vi "Teleop.vi"(10 "Match Info":T2={"Autonomous Elapsed Seconds"=0.0, "TeleOp Elapsed Seconds"=0.0, "Disabled Elapsed Seconds"=0.0, "Visited Autonomous"=FALSE, "Visited TeleOp"=FALSE, "Visited Disabled"=FALSE, "Autonomous Settings"={"Autonomous Style"=enum."Independent", "VI Refnum"=refnum}}, 11 "Call Context":T3) -> ()   [LabVIEW 2018]
doc: "This VI is called for each TeleOp packet received from the DS where the robot is not disabled. It is often used to read from the joysticks and update I/O or to update setpoints for timed control loops. It should complete and return within 20 milliseconds or it may miss DS packets."
uses:
  <vilib>/Rock Robotics/WPI/DriverStation/WPI_DriverStationDerivedRobotMode.ctl
  <vilib>/Rock Robotics/WPI/DriverStation/WPI_DriverStationMatch Info.ctl
  <vilib>/Rock Robotics/WPI/ThirdParty/Phoenix-LabVIEW/Motor Controller/Controls/CTRE_Phoenix_MotorControl_ControlMode.ctl
  <vilib>/Rock Robotics/Network Tables/NT Read Boolean.vi
  <vilib>/Rock Robotics/Network Tables/NT Read Number.vi
  <vilib>/Rock Robotics/WPI/Utilities/WPI_GetSetVariantRefNum.vi
  <vilib>/Rock Robotics/Network Tables/NT Write Boolean Array.vi
  <vilib>/Rock Robotics/Network Tables/NT Write Numeric Array.vi
  <vilib>/Rock Robotics/Network Tables/NT Write Boolean.vi
  <vilib>/Rock Robotics/Network Tables/NT Write Number.vi
  <vilib>/Rock Robotics/WPI/ThirdParty/Phoenix-LabVIEW/Motor Controller/Get/CTRE_Phoenix_MotorController_GetVoltage.vi
  <vilib>/Rock Robotics/WPI/ThirdParty/Phoenix-LabVIEW/Motor Controller/Get/CTRE_Phoenix_MotorController_GetSelectedSensorData.vi
  <vilib>/Rock Robotics/WPI/ThirdParty/Phoenix-LabVIEW/Motor Controller/Get/CTRE_Phoenix_MotorController_GetOutputCurrent_Enhanced.vi
  <vilib>/addons/control/pid/NI_PID_pid.lvlib
  Robot Global Data.vi
  <vilib>/addons/control/pid/pid.llb/PID (DBL).vi
panel:
  in  "Lift Position":i32=10000
  out "Button X 2":bool
  out "Button BACK 2":bool
  out "Button RT 2":bool
  out "Button LT 2":bool
  out "Button RB 2":bool
  out "Button LB 2":bool
  out "Button Y 2":bool
  out "Button B 2":bool
  out "Button A 2":bool
  in  "Right Max Acceleration (per 100ms)":i32=18000
  in  "Right Cruise Velocity (per 100 ms)":i32=20000
  out "Right Velocity per 100 ms":i32(graph)
  out "Right Position New 180":i32
  out "Right Position old":i32
  in  "Left Max Acceleration (per 100ms)":i32=18000
  in  "Left Cruise Velocity (per 100 ms)":i32=20000
  out "Left Velocity per 100 ms":i32(graph)
  out "Button Pressed?":bool
  out "Left Position New 180":i32
  out "Left Position old":i32
  out "Button X":bool
  out "Button BACK":bool
  out "Button RT":bool
  out "Button LT":bool
  out "Button RB":bool
  out "Button LB":bool
  out "Button Y":bool
  out "Button B":bool
  out "Button A":bool
  out "Wrist Position":i32=2000
  in  "Wrist Position":i32=10000 min=0 max=450000 step=50000
  out "Percent Output":dbl(graph)
  out "Position (Raw Sensor Units)":i32(graph)
  out "Velocity (Raw Sensor Units per 100 ms)":i32(graph)
  out "Elevator Position":i32=2000
  in  "Elevator Height":i32=10000 min=0 max=200000 step=10000
  out "Percent Output Elevator":dbl(graph)
  out "Position (Raw Sensor Units) 2":i32(graph)
  out "Velocity (Raw Sensor Units per 100 ms) 2":i32(graph)
  out "Output Current":dbl(graph)
  in  "Square Inputs":bool=TRUE
  in  "Gyro Rotation \nControl Enable?":bool
  in  "PID gains":T1={"proportional gain (Kc)"=0.02, "integral time (Ti, min)"=0.0, "derivative time (Td, min)"=0.0}
  in  "output range":cluster{"output high":dbl, "output low":dbl}={"output high"=0.6, "output low"=-0.6}
  out "Sample Slider 0":dbl(slide) scale=0.0..5.0
  out "Sample Boolean 1":bool
  out "Sample Boolean 0":bool
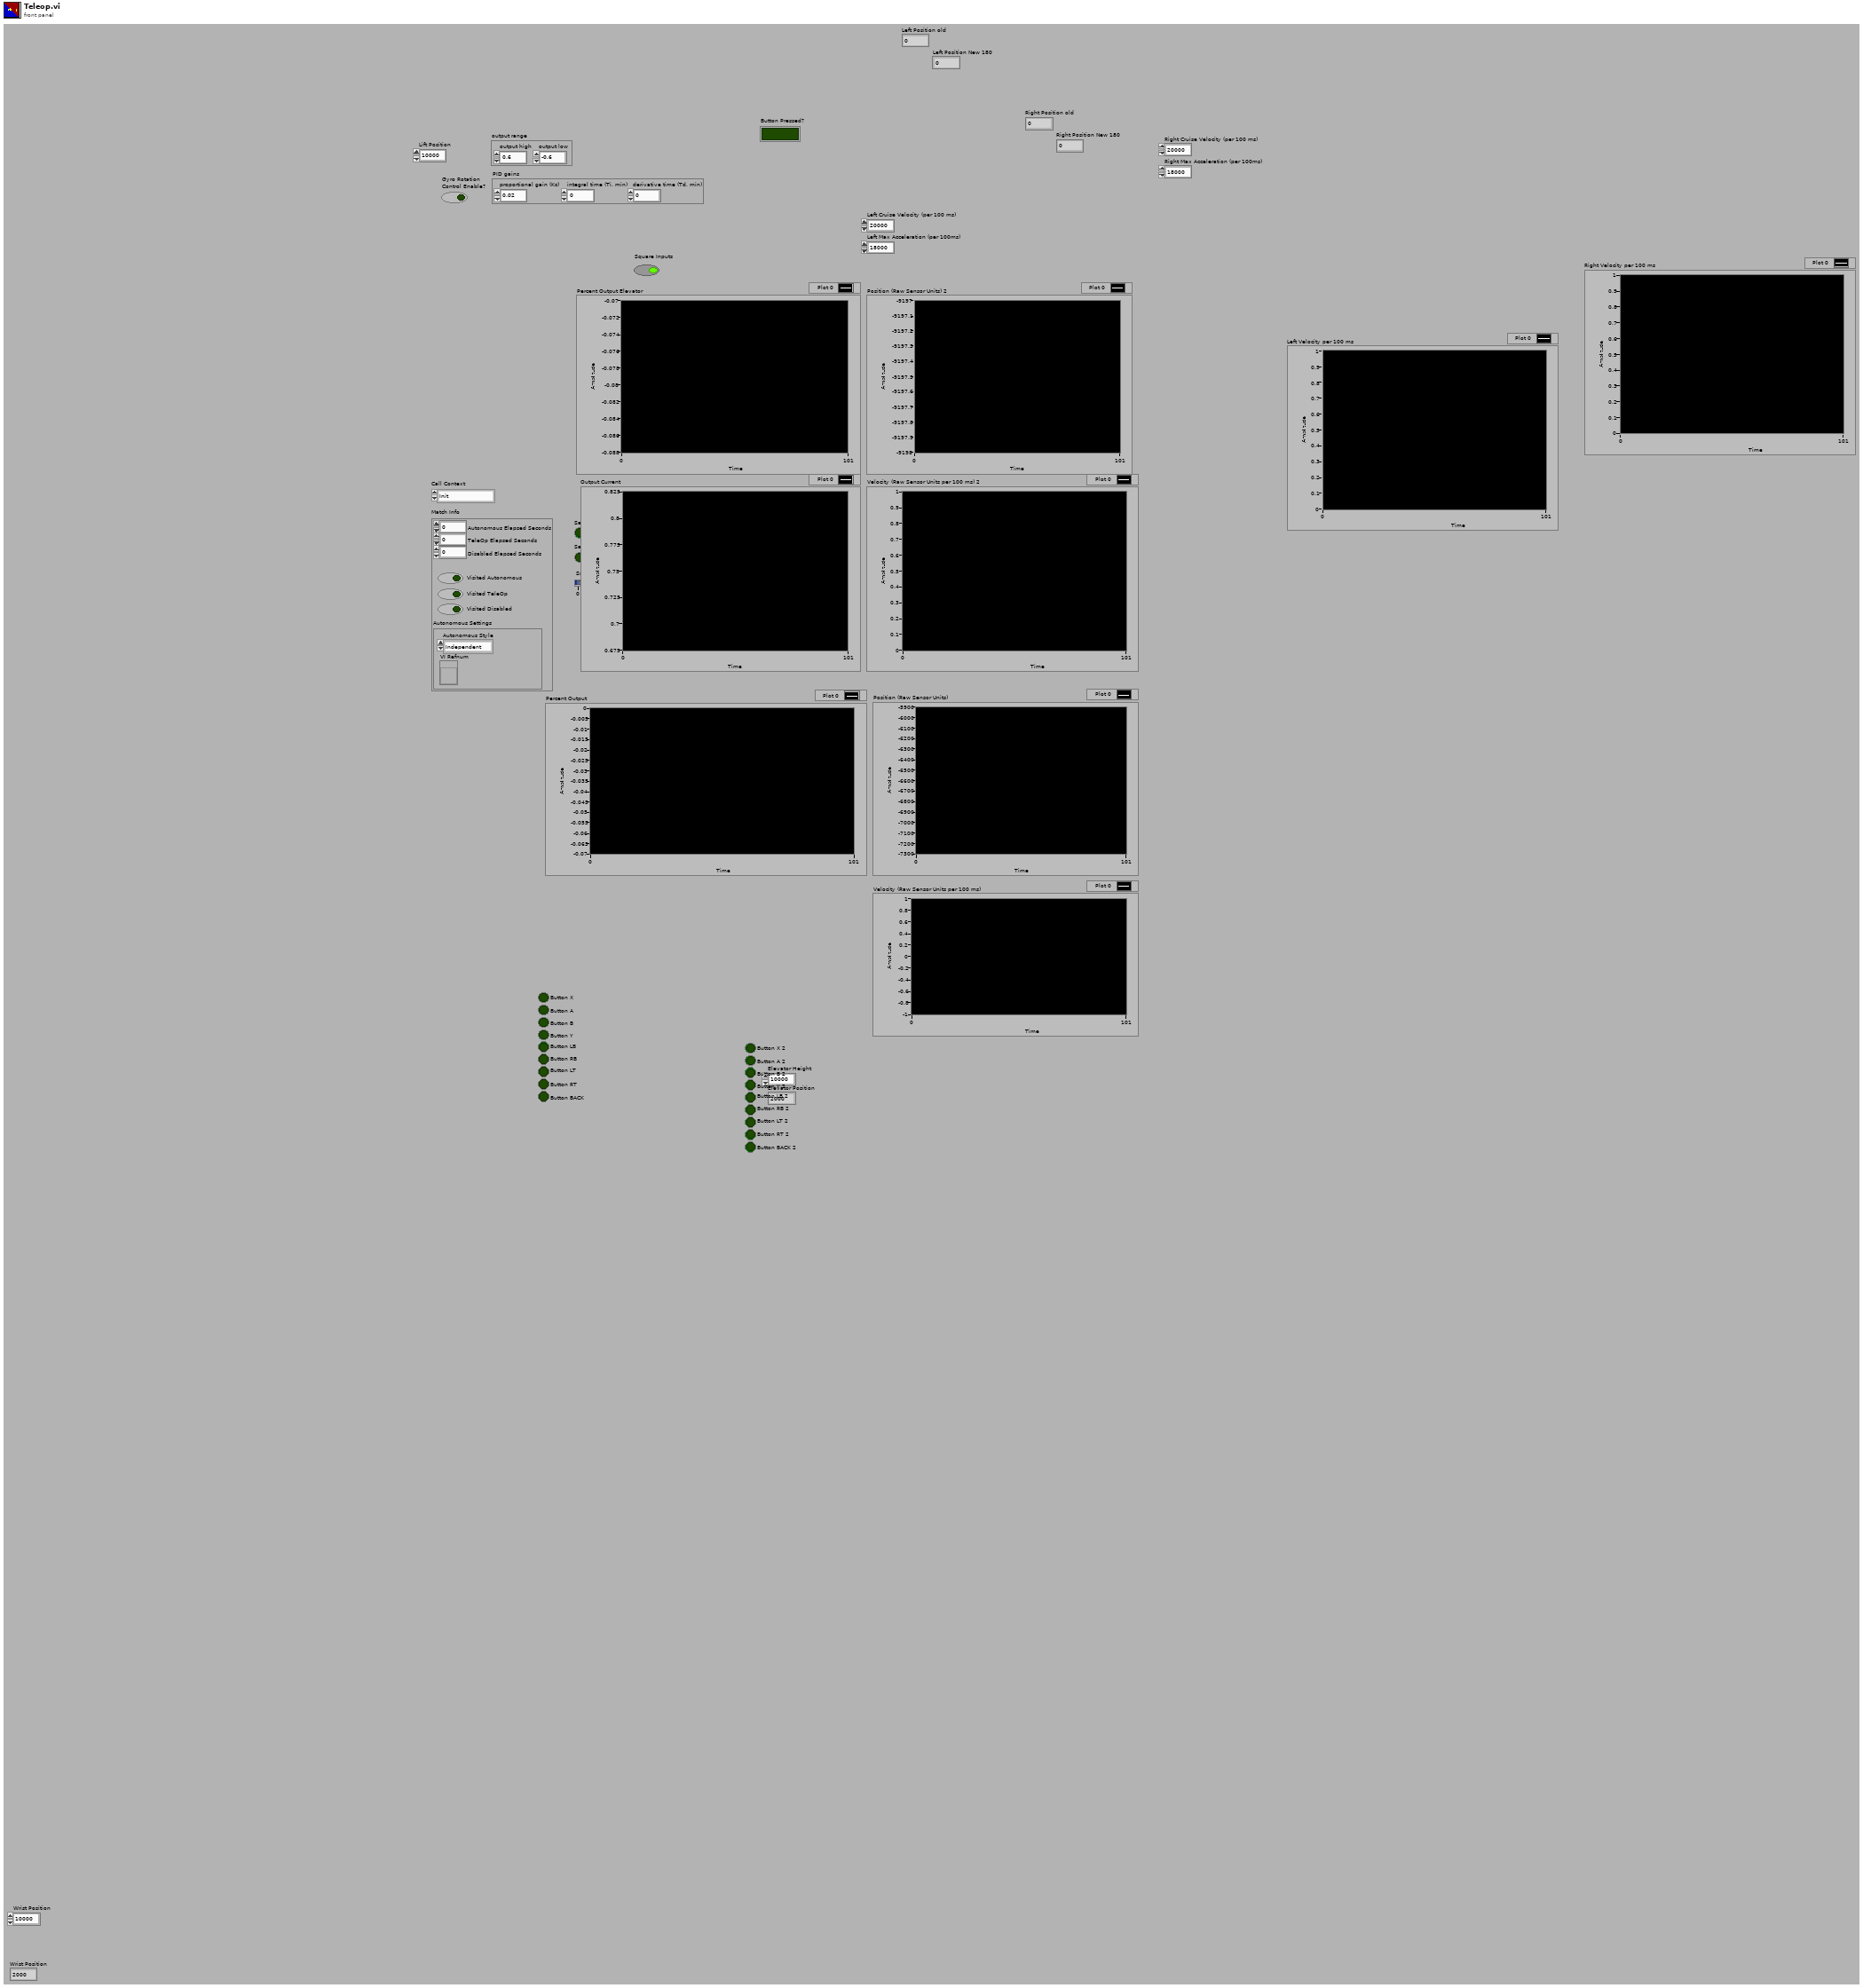
[diagram p1: front panel]
types:
  T1 = cluster{"proportional gain (Kc)":dbl, "integral time (Ti, min)":dbl, "derivative time (Td, min)":dbl}
  T2 = typedef "WPI_DriverStationMatch Info.ctl" = cluster{"Autonomous Elapsed Seconds":dbl, "TeleOp Elapsed Seconds":dbl, "Disabled Elapsed Seconds":dbl, "Visited Autonomous":bool, "Visited TeleOp":bool, "Visited Disabled":bool, "Autonomous Settings":cluster{"Autonomous Style":enum16{"Iterative", "Independent"}, "VI Refnum":refnum<vi>}}
  T3 = typedef "WPI_DriverStationDerivedRobotMode.ctl" = enum16{"Init", "Execute", "Stop"}
  T4 = typedef "CTRE_Phoenix_MotorControl_ControlMode.ctl" = u16
  T5 = typedef "WPI_JoystickDevRef.ctl" = cluster{"Device":T6}
  T6 = typedef "WPI_JoystickDeviceEnum.ctl" = enum16{"USB 0", "USB 1", "USB 2", "USB 3", "USB 4", "USB 5"}
  T7 = cluster{"Buttons[0]":bool, "Buttons[1]":bool, "Buttons[2]":bool, "Buttons[3]":bool, "Buttons[4]":bool, "Buttons[5]":bool, "Buttons[6]":bool, "Buttons[7]":bool, "Buttons[8]":bool}
  T8 = typedef "WPI_GyroDevRef.ctl" = cluster{"DevStatus":errorcluster, "Analog Channel":T9, "Gain (VoltsPerDegree/Second)":dbl, "Gyro Type":enum16{"Analog", "XRS450"}, "Handle":i32, "SPI Bus":T10, "Device Found":bool, "Sample Rate":dbl, "Calibrate On Open":bool, "Offset":dbl}
  T9 = typedef "FPGA_AIChannel.ctl" = enum8{"AI 0", "AI 1", "AI 2", "AI 3", "AI MXP 0", "AI MXP 1", "AI MXP 2", "AI MXP 3", "Invalid"}
  T10 = typedef "spi_bus.ctl" = enum16{"SPI On-Board, CS0", "SPI On-Board, CS1", "SPI On-Board, CS2", "SPI On-Board, CS3", "SPI MXP", "Invalid"}
  T11 = typedef "WPI_MotorControlDeviceRef.ctl" = cluster{"DeviceStatus":errorcluster, "Type":T12, "PWM":cluster{"PWM Channel":T13, "DeadBand":T14}, "CAN":cluster{"Device Number":u8, "SetOutput VI Ref":variant, "GetOutput VI Ref":variant, "Enable VI Ref":variant, "Disable VI Ref":variant, "Data":variant}, "Invert":bool, "DIO PWM":cluster{"PWM \"Enable\" Channel":T13, "DIOChannel":T15, "PWM Rate":dbl}}
  T12 = typedef "WPI_MotorControlType.ctl" = enum16{"PWM", "CAN", "DIO PWM"}
  T13 = typedef "FPGA_DIOPWMChannel.ctl" = enum8{"PWM 0", "PWM 1", "PWM 2", "PWM 3", "PWM 4", "PWM 5", "PWM 6", "PWM 7", "PWM 8", "PWM 9", "PWM MXP 0", "PWM MXP 1", "PWM MXP 2", "PWM MXP 3", "PWM MXP 4", "PWM MXP 5", "PWM MXP 6", "PWM MXP 7", "PWM MXP 8", "PWM MXP 9", "Invalid"}
  T14 = typedef "WPI_PWMDeadband.ctl" = cluster{"Name":string, "maxPositivePwm":i32, "minPositivePwm":i32, "centerPwm":i32, "maxNegativePwm":i32, "minNegativePwm":i32, "angularRange":u16}
  T15 = typedef "FPGA_DIOChannel.ctl" = enum8{"DIO 0", "DIO 1", "DIO 2", "DIO 3", "DIO 4", "DIO 5", "DIO 6", "DIO 7", "DIO 8", "DIO 9", "DIO MXP 0", "DIO MXP 1", "DIO MXP 2", "DIO MXP 3", "DIO MXP 4", "DIO MXP 5", "DIO MXP 6", "DIO MXP 7", "DIO MXP 8", "DIO MXP 9", "DIO MXP 10", "DIO MXP 11", "DIO MXP 12", "DIO MXP 13", "DIO MXP 14", "DIO MXP 15", "SPI Port CS1", "SPI Port CS2", "SPI Port CS3", "SPI Port MISO", "SPI Port MOSI", "Invalid"}
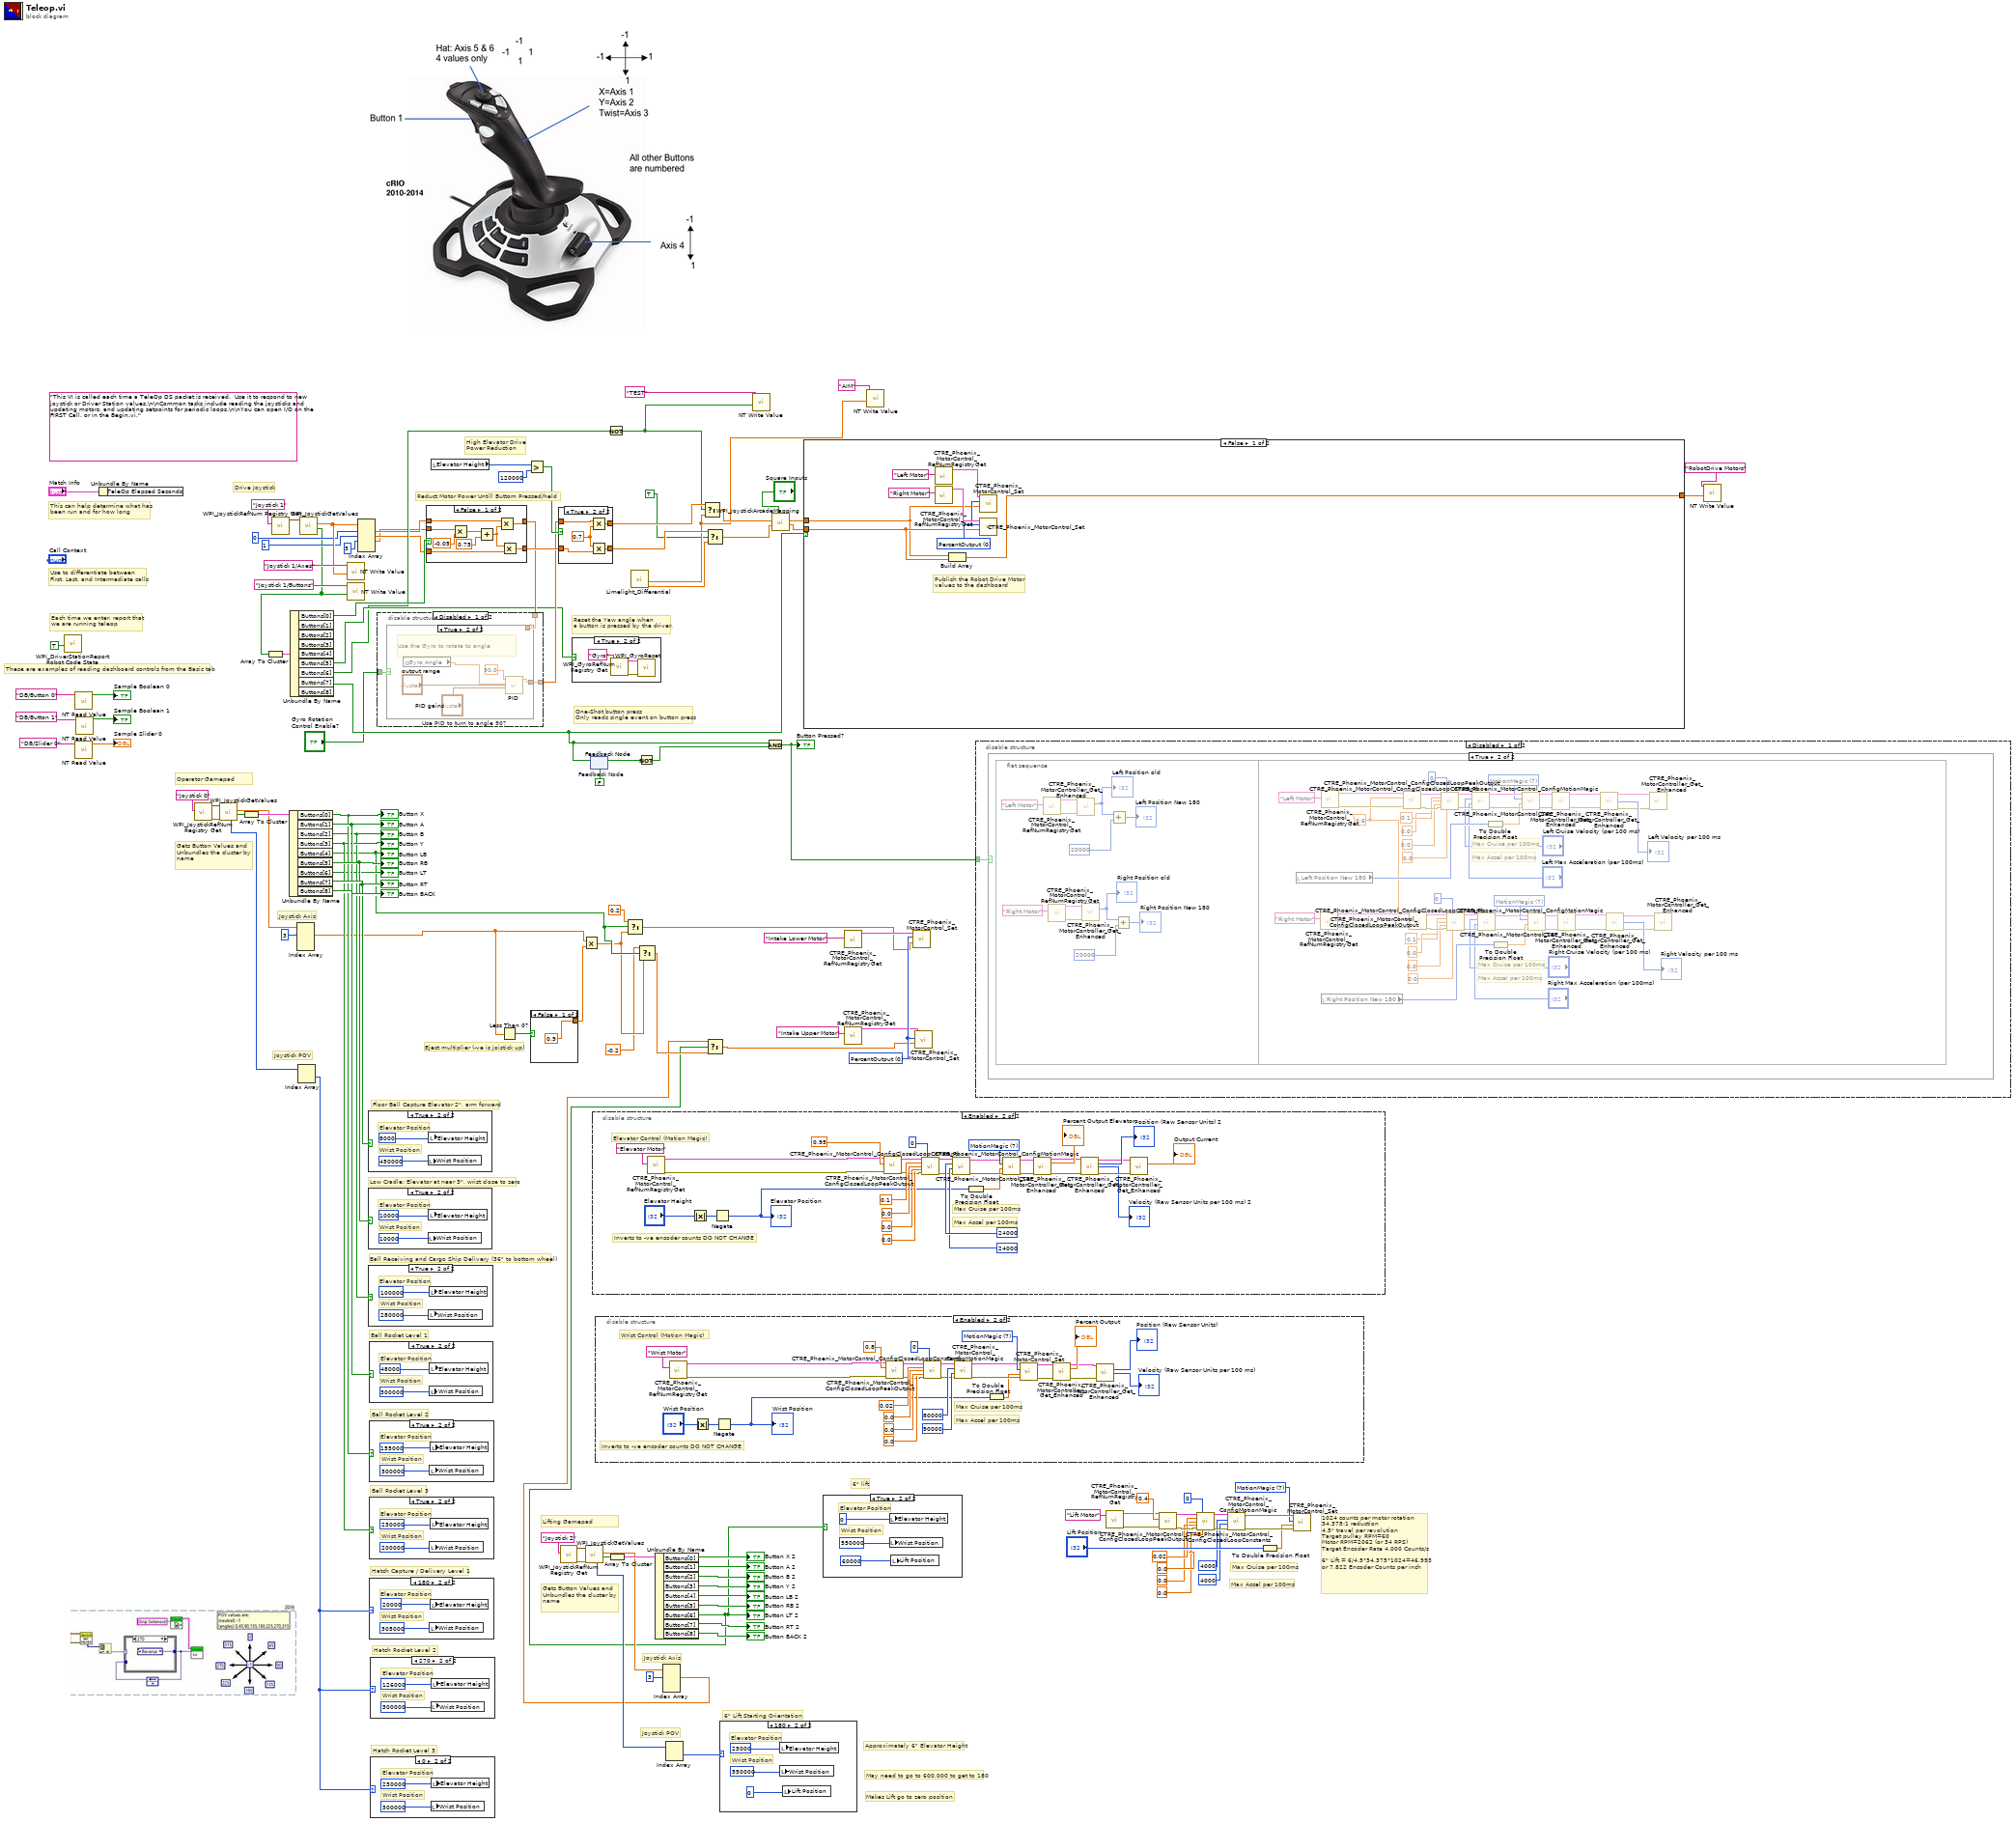
[diagram p0: block diagram]
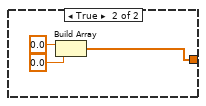
[diagram p8: hidden frame]
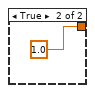
[diagram p9: hidden frame]
diagram:
  w4 = T4 7 items=["PercentOutput"=0, "Position"=1, "Velocity"=2, "Current"=3, "Follower"=5, "MotionProfile"=6, "MotionMagic"=7, "MotionProfileArc"=10, "Disabled"=15] ("Wrist Control Mode")
  w74 = T4 0 items=["PercentOutput"=0, "Position"=1, "Velocity"=2, "Current"=3, "Follower"=5, "MotionProfile"=6, "MotionMagic"=7, "MotionProfileArc"=10, "Disabled"=15] ("Control Mode")
  (unwired) "This VI is called each time a TeleOp DS packet is received.  Use it to respond to new joystick or Driver Station values.\n\nCommon tasks include reading the joysticks and updating motors, and updating setpoints for periodic loops.\n\nYou can open I/O on the FIRST Call, or in the Begin.vi."
  # "6\" lift"
  # "1024 counts per motor rotation\n34.375:1 reduction\n4.5\" travel per revolution\nTarget pulley RPM=60\nMotor RPM=2062 (or 34 RPS)\nTarget Encoder Rate 4,000 Counts/s\n\n6\" Lift = 6/4.5*34.375*1024=46,993\nor 7,822 Encoder Counts per inch"
  # "Max Accel per 100ms"
  # "Max Cruise per 100ms"
  # "Makes Lift go to zero position"
  # "Approximately 6\" Elevator Height"
  # "May need to go to 600,000 to get to 180"
  # "6\" Lift Starting Orientation"
  # "Joystick POV"
  # "Joystick Axis"
  # "Lifting Gamepad"
  # "Gets Button Values and Unbundles the cluster by name"
  # "One-Shot button press \nOnly reads single event on button press"
  # "Eject multiplier (-ve is joistick up)"
  # "Ball Rocket Level 3"
  # "Hatch Rocket Level 2"
  # "Joystick POV"
  # "Hatch Rocket Level 3"
  # "Hatch Capture / Delivery Level 1"
  # "Ball Rocket Level 2"
  # "Ball Rocket Level 1"
  # "Ball Receiving and Cargo Ship Delivery (36\" to bottom wheel)"
  # "Low Cradle: Elevator at near 3\", wrist close to zero"
  # "Floor Ball Capture Elevator 2\", arm forward"
  # "Joystick Axis"
  # "Operator Gamepad"
  # "Gets Button Values and Unbundles the cluster by name"
  # "Reset the Yaw angle when \na button is pressed by the driver."
  # "High Elevator Drive \nPower Reduction"
  # "Reduct Motor Power Untill Buttom Pressed/held"
  # "Drive Joystick"
  # "These are examples of reading dashboard controls from the Basic tab"
  # "Each time we enter, report that\nwe are running teleop"
  # "Use to differentiate between\nFirst, Last, and Intermediate calls"
  # "This can help determine what has\nbeen run and for how long"
  n1 = call <vilib>:"WPI_DriverStationReport Robot Code State.vi"("TeleOp"=TRUE ("Autonomous")) -> ()  [unwired: 10 in, 1 out]
  n2 = call-poly <vilib>:"NT Read Value.vi"("Name"="DB/Button 0" ("refnum name")) -> ("Boolean"=→"Sample Boolean 0":bool)  [unwired: 9 in, 1 out]
  n3 = call-poly <vilib>:"NT Read Value.vi"("Name"="DB/Slider 0" ("refnum name")) -> ("Numeric"=→"Sample Slider 0":dbl)  [unwired: 9 in, 1 out]
  n4 = call-poly <vilib>:"NT Read Value.vi"("Name"="DB/Button 1" ("refnum name")) -> ("Boolean"=→"Sample Boolean 1":bool)  [unwired: 9 in, 1 out]
  n5 = Unbundle By Name("Match Info") -> ()  [unwired: 1 out]
  n6 = call <vilib>:"WPI_JoystickRefNum Registry Get.vi"("refnum name"="Joystick 0") -> ("error out"=w87:errorcluster, "JoystickDevRef"=w88:T5)  [unwired: 1 in, 8 out]
  n7 = call <vilib>:"WPI_JoystickGetValues.vi"("error in (no error)"=w87, "JoystickDevRef"=w88) -> ("Buttons"=w84:bool[], "Axes"=w86:dbl[], "POVs"=w85:i16[])  [unwired: 5 in, 2 out]
  n8 = Array To Cluster(array=w84) -> (cluster=w94:T7)
  n9 = call <vilib>:"WPI_JoystickRefNum Registry Get.vi"("refnum name"="Joystick 1") -> ("JoystickDevRef"=w113:T5)  [unwired: 1 in, 9 out]
  n10 = Unbundle By Name(w94) -> ("Buttons[0]"=w82:bool, "Buttons[1]"=w83:bool, "Buttons[2]"=w80:bool, "Buttons[3]"=w81:bool, "Buttons[4]"=w77:bool, "Buttons[5]"=w90:bool, "Buttons[6]"=→"Button LT":bool, "Buttons[7]"=w91:bool, "Buttons[8]"=→"Button BACK":bool)
  "Button A" <- w83
  "Button B" <- w80
  "Button Y" <- w81
  "Button LB" <- w77
  "Button RB" <- w90
  "Button RT" <- w91
  "Button X" <- w82
  n11 = Index Array(array=w86, index #1=3 ("index")) -> (element #1=w78:dbl)  [unwired: 3 in, 3 out]
  n12 = Index Array(array=w85) -> (element #1=w89:i16)  [unwired: 2 in, 1 out]
  n13 = call <vilib>:"WPI_JoystickGetValues.vi"("JoystickDevRef"=w113) -> ("Buttons"=w102:bool[], "Axes"=w110:dbl[])  [unwired: 6 in, 3 out]
  n14 = Array To Cluster(array=w102) -> (cluster=w104:T7)
  n15 = Unbundle By Name(w104) -> ("Buttons[0]"=w103:bool, "Buttons[5]"=w99:bool, "Buttons[6]"=w54:bool, "Buttons[7]"=w61:bool)  [unwired: 5 out]
  n16 = call-poly <vilib>:"NT Write Value.vi"("Numeric Array"=w110, "Name"="Joystick 1/Axes") -> ()  [unwired: 9 in, 1 out]
  n17 = call-poly <vilib>:"NT Write Value.vi"("Boolean Array"=w102, "Name"="Joystick 1/Buttons") -> ()  [unwired: 9 in, 1 out]
  n18 = Index Array(array=w110, index #1=0 ("index"), index #2=1 ("index"), index #3=3 ("index")) -> (element #1=w53:dbl, element #2=w52:dbl, element #3=w42:dbl)  [unwired: 2 in, 2 out]
  n19 = case shown="True" w91 {
    frame False {
    }
    frame True {
      # "Wrist Position"
      # "Elevator Position"
      n20 = local write "Wrist Position"(450000) -> ()
      n21 = local write "Elevator Height"(8000) -> ()
    }
  }
  n22 = case shown="True" w90 {
    frame False {
    }
    frame True {
      # "Wrist Position"
      # "Elevator Position"
      n23 = local write "Wrist Position"(10000) -> ()
      n24 = local write "Elevator Height"(10000) -> ()
    }
  }
  n25 = case shown="True" w80 {
    frame False {
    }
    frame True {
      # "Wrist Position"
      # "Elevator Position"
      n26 = local write "Wrist Position"(280000) -> ()
      n27 = local write "Elevator Height"(100000) -> ()
    }
  }
  n28 = case shown="True" w83 {
    frame False {
    }
    frame True {
      # "Wrist Position"
      # "Elevator Position"
      n29 = local write "Wrist Position"(300000) -> ()
      n30 = local write "Elevator Height"(48000) -> ()
    }
  }
  n31 = case shown="True" w82 {
    frame False {
    }
    frame True {
      # "Wrist Position"
      # "Elevator Position"
      n32 = local write "Wrist Position"(300000) -> ()
      n33 = local write "Elevator Height"(155000) -> ()
    }
  }
  n34 = case shown="True" w81 {
    frame False {
    }
    frame True {
      # "Wrist Position"
      # "Elevator Position"
      n35 = local write "Wrist Position"(200000) -> ()
      n36 = local write "Elevator Height"(230000) -> ()
    }
  }
  n37 = case shown="180" w89 {
    frame -1, Default {
    }
    frame 180 {
      # "Wrist Position"
      # "Elevator Position"
      n38 = local write "Wrist Position"(305000) -> ()
      n39 = local write "Elevator Height"(20000) -> ()
    }
  }
  n40 = case shown="270" w89 {
    frame -1, Default {
    }
    frame 270 {
      # "Wrist Position"
      # "Elevator Position"
      n41 = local write "Wrist Position"(300000) -> ()
      n42 = local write "Elevator Height"(126000) -> ()
    }
  }
  n43 = case shown="0" w89 {
    frame -1, Default {
    }
    frame 0 {
      # "Wrist Position"
      # "Elevator Position"
      n44 = local write "Wrist Position"(300000) -> ()
      n45 = local write "Elevator Height"(230000) -> ()
    }
  }
  n46 = case shown="False" w103 {
    tunnel: [w148 w154] -> w101
    tunnel: [w149 w152] -> w105
    tunnel: w53 -> [w147 w151]
    tunnel: w52 -> [w146 w150]
    tunnel: w42 -> [w145 _]
    frame False {
      n47 = Multiply(x=w145, y=-0.05 ("drive multiplyer")) -> (x*y=w143:dbl)
      n48 = Add(x=w143, y=0.75 ("drive multiplyer")) -> (x+y=w141:dbl)
      n49 = Multiply(x=w147, y=w141) -> (x*y=w148:dbl)
      n50 = Multiply(x=w141, y=w146) -> (x*y=w149:dbl)
    }
    frame True {
      w153 = 1.0
      n51 = Multiply(x=w151, y=w153) -> (x*y=w154:dbl)
      n52 = Multiply(x=w153, y=w150) -> (x*y=w152:dbl)
    }
  }
  n53 = disable-structure shown="Disabled" {
    disable-tunnel: w101 -> [w157 _]
    disable-tunnel: [w156 _] -> w100
    disable-tunnel: "Gyro Rotation \nControl Enable?" -> [w155 _]
    frame Disabled {
      n54 = case "Use PID to turn to angle 90?" shown="True" w155 {
        tunnel: [w158 w160] -> w156
        tunnel: w157 -> [w158 _]
        frame False {
        }
        frame True {
          # "Use the Gyro to rotate to angle"
          n55 = global read "Robot Global Data.vi" "Gyro Angle"() -> (w159:dbl)
          n56 = call-poly <vilib>:"PID.vi"("output range"="output range", "PID gains"="PID gains", "process variable"=w159, "setpoint"=90.0) -> ("output"=w160:dbl)  [unwired: 6 in, 1 out]
        }
      }
    }
    frame Enabled {
    }
  }
  n57 = local read "Elevator Height"() -> (w65:i32)
  n58 = Less Than 0?(x=w78) -> (x < 0?=w66:bool)
  n59 = Greater?(x=w65, y=120000) -> (0:w106:bool)
  n60 = case shown="False" w66 {
    tunnel: [0.9 1.0] -> w70
    frame False {
    }
    frame True {
    }
  }
  n61 = case shown="True" w106 {
    tunnel: w100 -> [w167 w171]
    tunnel: w105 -> [w166 w170]
    tunnel: [w167 w169] -> w47
    tunnel: [w166 w168] -> w48
    frame False {
    }
    frame True {
      w172 = 0.7
      n62 = Multiply(x=w171, y=w172) -> (x*y=w169:dbl)
      n63 = Multiply(x=w172, y=w170) -> (x*y=w168:dbl)
    }
  }
  n64 = call <vilib>:"WPI_JoystickRefNum Registry Get.vi"("refnum name"="Joystick 2") -> ("error out"=w35:errorcluster, "JoystickDevRef"=w36:T5)  [unwired: 1 in, 8 out]
  n65 = case shown="True" w99 {
    frame False {
    }
    frame True {
      n66 = call <vilib>:"WPI_GyroRefNum Registry Get.vi"("refnum name"="Gyro") -> ("error out"=w173:errorcluster, "GyroDevRef"=w174:T8)  [unwired: 9 in]
      n67 = call <vilib>:"WPI_GyroReset.vi"("error in"=w173, "GyroDevRef"=w174) -> ()  [unwired: 8 in, 2 out]
    }
  }
  n68 = Multiply(x=w78, y=w70) -> (x*y=w71:dbl)
  n69 = call <vilib>:"WPI_JoystickGetValues.vi"("error in (no error)"=w35, "JoystickDevRef"=w36) -> ("Buttons"=w33:bool[], "Axes"=w34:dbl[], "POVs"=w27:i16[])  [unwired: 5 in, 2 out]
  n70 = feedback #1 "Feedback Node"(FALSE ("Button In")) -> (w64:bool)
  n71 = feedback-in #1(w61) -> ()
  n72 = disable-structure shown="Enabled" {
    frame Disabled {
    }
    frame Enabled {
      w196 = T4 7 items=["PercentOutput"=0, "Position"=1, "Velocity"=2, "Current"=3, "Follower"=5, "MotionProfile"=6, "MotionMagic"=7, "MotionProfileArc"=10, "Disabled"=15] ("Elevator Control Mode")
      # "Max Accel per 100ms"
      # "Max Cruise per 100ms"
      # "Inverts to -ve encoder counts DO NOT CHANGE"
      # "Elevator Control (Motion Magic)"
      n73 = call <vilib>:"CTRE_Phoenix_MotorControl_RefNumRegistryGet.vi"("refnum name"="Elevator Motor") -> ("error out"=w186:errorcluster, "PhoenixMotorControlDevRef"=w187:T11)  [unwired: 9 in]
      n74 = Absolute Value(x="Elevator Height") -> (abs(x)=w195:i32)
      n75 = Negate(x=w195) -> (-x=w188:i32)
      "Elevator Position" <- w188
      n76 = call <vilib>:"CTRE_Phoenix_MotorControl_ConfigClosedLoopPeakOutput.vi"("error in (no error)"=w186, "peakOutput"=0.95 ("Peak Elevator Power"), "PhoenixMotorControlDevRef"=w187) -> ("error out"=w192:errorcluster, "PhoenixMotorControlDevRef"=w205:T11)  [unwired: 7 in]
      n77 = call <vilib>:"CTRE_Phoenix_MotorControl_ConfigClosedLoopConstants.vi"("PhoenixMotorControlDevRef"=w205, "slotIdx"=0, "P"=0.1 ("P 2"), "I"=0.0 ("I 2"), "D"=0.0 ("D 2"), "error in (no error)"=w192, "F"=0.0 ("F 2")) -> ("PhoenixMotorControlDevRef"=w200:T11, "error out"=w191:errorcluster)  [unwired: 7 in]
      n78 = call <vilib>:"CTRE_Phoenix_MotorControl_ConfigMotionMagic.vi"("error in (no error)"=w191, "Acceleration"=24000 ("Elevator Max Acceleration (per 100ms)"), "Cruise Velocity"=24000 ("Elevator Cruise Velocity (per 100 ms)"), "PhoenixMotorControlDevRef"=w200) -> ("error out"=w190:errorcluster, "PhoenixMotorControlDevRef"=w193:T11)  [unwired: 6 in]
      n79 = To Double Precision Float(number=w188) -> (double precision float=w189:dbl)
      n80 = call <vilib>:"CTRE_Phoenix_MotorControl_Set.vi"("error in (no error)"=w190, "Output"=w189, "Control Mode"=w196, "PhoenixMotorControlDevRef"=w193) -> ("error out"=w184:errorcluster, "PhoenixMotorControlDevRef"=w185:T11)  [unwired: 6 in]
      n81 = call-poly <vilib>:"CTRE_Phoenix_MotorController_Get_Enhanced.vi"("PhoenixMotorControlDevRef"=w185, "error in"=w184) -> ("PhoenixMotorControlDevRef"=w182:T11, "Percent Output"=→"Percent Output Elevator":dbl, "error out"=w181:errorcluster)  [unwired: 9 in, 2 out]
      n82 = call-poly <vilib>:"CTRE_Phoenix_MotorController_Get_Enhanced.vi"("PhoenixMotorControlDevRef"=w182, "error in"=w181) -> ("PhoenixMotorControlDevRef"=w179:T11, "Position (Raw Sensor Units)"=→"Position (Raw Sensor Units) 2":i32, "Velocity (Raw Sensor Units per 100 ms)"=→"Velocity (Raw Sensor Units per 100 ms) 2":i32, "error out"=w178:errorcluster)  [unwired: 10 in]
      n83 = call-poly <vilib>:"CTRE_Phoenix_MotorController_Get_Enhanced.vi"("PhoenixMotorControlDevRef"=w179, "error in"=w178) -> ("Output Current"=→"Output Current":dbl)  [unwired: 11 in, 2 out]
    }
  }
  n84 = disable-structure shown="Enabled" {
    frame Disabled {
    }
    frame Enabled {
      w225 = T4 7 items=["PercentOutput"=0, "Position"=1, "Velocity"=2, "Current"=3, "Follower"=5, "MotionProfile"=6, "MotionMagic"=7, "MotionProfileArc"=10, "Disabled"=15] ("Wrist Control Mode")
      # "Max Accel per 100ms"
      # "Max Cruise per 100ms"
      # "Inverts to -ve encoder counts DO NOT CHANGE"
      # "Wrist Control (Motion Magic)"
      n85 = call <vilib>:"CTRE_Phoenix_MotorControl_RefNumRegistryGet.vi"("refnum name"="Wrist Motor") -> ("error out"=w215:errorcluster, "PhoenixMotorControlDevRef"=w216:T11)  [unwired: 9 in]
      n86 = Absolute Value(x="Wrist Position") -> (abs(x)=w224:i32)
      n87 = Negate(x=w224) -> (-x=w218:i32)
      "Wrist Position" <- w218
      n88 = call <vilib>:"CTRE_Phoenix_MotorControl_ConfigClosedLoopPeakOutput.vi"("error in (no error)"=w215, "peakOutput"=0.8 ("Peak Wrist Power"), "PhoenixMotorControlDevRef"=w216) -> ("error out"=w221:errorcluster, "PhoenixMotorControlDevRef"=w234:T11)  [unwired: 7 in]
      n89 = call <vilib>:"CTRE_Phoenix_MotorControl_ConfigClosedLoopConstants.vi"("PhoenixMotorControlDevRef"=w234, "slotIdx"=0, "P"=0.02 ("P 3"), "I"=0.0 ("I 3"), "D"=0.0 ("D 3"), "error in (no error)"=w221, "F"=0.0 ("F 3")) -> ("PhoenixMotorControlDevRef"=w229:T11, "error out"=w220:errorcluster)  [unwired: 7 in]
      n90 = call <vilib>:"CTRE_Phoenix_MotorControl_ConfigMotionMagic.vi"("error in (no error)"=w220, "Acceleration"=90000 ("Wrist Max Acceleration"), "Cruise Velocity"=80000 ("Wrist Cruise Velocity"), "PhoenixMotorControlDevRef"=w229) -> ("error out"=w219:errorcluster, "PhoenixMotorControlDevRef"=w222:T11)  [unwired: 6 in]
      n91 = To Double Precision Float(number=w218) -> (double precision float=w217:dbl)
      n92 = call <vilib>:"CTRE_Phoenix_MotorControl_Set.vi"("error in (no error)"=w219, "Output"=w217, "Control Mode"=w225, "PhoenixMotorControlDevRef"=w222) -> ("error out"=w213:errorcluster, "PhoenixMotorControlDevRef"=w214:T11)  [unwired: 6 in]
      n93 = call-poly <vilib>:"CTRE_Phoenix_MotorController_Get_Enhanced.vi"("PhoenixMotorControlDevRef"=w214, "error in"=w213) -> ("PhoenixMotorControlDevRef"=w211:T11, "Percent Output"=→"Percent Output":dbl, "error out"=w210:errorcluster)  [unwired: 9 in, 2 out]
      n94 = call-poly <vilib>:"CTRE_Phoenix_MotorController_Get_Enhanced.vi"("PhoenixMotorControlDevRef"=w211, "error in"=w210) -> ("Position (Raw Sensor Units)"=→"Position (Raw Sensor Units)":i32, "Velocity (Raw Sensor Units per 100 ms)"=→"Velocity (Raw Sensor Units per 100 ms)":i32)  [unwired: 10 in, 2 out]
    }
  }
  n95 = Not(x=w54) -> (.not. x?=w46:bool)
  n96 = Array To Cluster(array=w33) -> (cluster=w40:T7)
  n97 = Select(t=0.2 ("Numeric"), s=w77, f=w71) -> (s? t:f=w67:dbl)
  n98 = call "Limelight_Differential.vi"() -> ("DriveCommand"=w49:dbl, "SteerCommand"=w45:dbl)  [unwired: 8 in, 1 out]
  n99 = Not(x=w64) -> (.not. x?=w63:bool)
  n100 = Select(t=-0.2 ("Numeric 2"), s=w77, f=w71) -> (s? t:f=w24:dbl)
  n101 = Unbundle By Name(w40) -> ("Buttons[0]"=→"Button X 2":bool, "Buttons[1]"=→"Button A 2":bool, "Buttons[2]"=→"Button B 2":bool, "Buttons[3]"=→"Button Y 2":bool, "Buttons[4]"=→"Button LB 2":bool, "Buttons[5]"=→"Button RB 2":bool, "Buttons[6]"=w21:bool, "Buttons[7]"=→"Button RT 2":bool, "Buttons[8]"=→"Button BACK 2":bool)
  "Button LT 2" <- w21
  n102 = Index Array(array=w34, index #1=3 ("index")) -> (element #1=w22:dbl)  [unwired: 3 in, 3 out]
  n103 = Index Array(array=w27) -> (element #1=w26:i16)  [unwired: 2 in, 1 out]
  n104 = Select(t=w47, s=w46, f=w45) -> (s? t:f=w51:dbl)
  n105 = Select(t=w48, s=TRUE, f=w49) -> (s? t:f=w50:dbl)
  n106 = Select(t=w22, s=w21, f=w24) -> (s? t:f=w23:dbl)
  n107 = case shown="180" w26 {
    frame -1, Default {
    }
    frame 180 {
      # "Wrist Position"
      # "Elevator Position"
      n108 = local write "Wrist Position"(550000) -> ()
      n109 = local write "Elevator Height"(25000) -> ()
      n110 = local write "Lift Position"(0) -> ()
    }
  }
  n111 = call-poly <vilib>:"NT Write Value.vi"("Boolean"=w46, "Name"="TEST") -> ()  [unwired: 9 in, 1 out]
  n112 = And(x=w61, y=w63) -> (x .and. y?=w60:bool)
  "Button Pressed?" <- w60
  n113 = call <vilib>:"WPI_JoystickArcadeMapping.vi"("Square Inputs"="Square Inputs", "Y axis value"=w50, "X axis value"=w51) -> ("Right Motor Value"=w97:dbl, "Left Motor Value"=w96:dbl)  [unwired: 7 in]
  n114 = case shown="False" w61 {
    tunnel: w97 -> [w242 _]
    tunnel: w96 -> [w241 _]
    tunnel: [w240 w248] -> w58
    frame False {
      w243 = T4 0 items=["PercentOutput"=0, "Position"=1, "Velocity"=2, "Current"=3, "Follower"=5, "MotionProfile"=6, "MotionMagic"=7, "MotionMagicArc"=8, "MotionProfileArc"=10, "Disabled"=15] ("Control Mode")
      # "Publish the Robot Drive Motor\nvalues to the dashboard"
      n115 = call <vilib>:"CTRE_Phoenix_MotorControl_RefNumRegistryGet.vi"("refnum name"="Left Motor") -> ("PhoenixMotorControlDevRef"=w245:T11)  [unwired: 9 in, 1 out]
      n116 = call <vilib>:"CTRE_Phoenix_MotorControl_RefNumRegistryGet.vi"("refnum name"="Right Motor") -> ("PhoenixMotorControlDevRef"=w244:T11)  [unwired: 9 in, 1 out]
      n117 = Build Array(w241, w242) -> (w240:dbl[])
      n118 = call <vilib>:"CTRE_Phoenix_MotorControl_Set.vi"("Output"=w241, "Control Mode"=w243, "PhoenixMotorControlDevRef"=w245) -> ()  [unwired: 7 in, 2 out]
      n119 = call <vilib>:"CTRE_Phoenix_MotorControl_Set.vi"("Output"=w242, "Control Mode"=w243, "PhoenixMotorControlDevRef"=w244) -> ()  [unwired: 7 in, 2 out]
    }
    frame True {
      n120 = Build Array(0.0 ("element"), 0.0 ("element")) -> (w248:dbl[])
    }
  }
  n121 = case shown="True" w21 {
    frame False {
    }
    frame True {
      # "Wrist Position"
      # "Elevator Position"
      n122 = local write "Elevator Height"(0) -> ()
      n123 = local write "Wrist Position"(550000) -> ()
      n124 = local write "Lift Position"(60000) -> ()
    }
  }
  n125 = call <vilib>:"CTRE_Phoenix_MotorControl_RefNumRegistryGet.vi"("refnum name"="Intake Lower Motor") -> ("PhoenixMotorControlDevRef"=w73:T11)  [unwired: 9 in, 1 out]
  n126 = call <vilib>:"CTRE_Phoenix_MotorControl_RefNumRegistryGet.vi"("refnum name"="Intake Upper Motor") -> ("PhoenixMotorControlDevRef"=w72:T11)  [unwired: 9 in, 1 out]
  n127 = call-poly <vilib>:"NT Write Value.vi"("Numeric"=w45, "Name"="AIM") -> ()  [unwired: 9 in, 1 out]
  n128 = call <vilib>:"CTRE_Phoenix_MotorControl_Set.vi"("Output"=w67, "Control Mode"=w74, "PhoenixMotorControlDevRef"=w73) -> ()  [unwired: 7 in, 2 out]
  n129 = call <vilib>:"CTRE_Phoenix_MotorControl_Set.vi"("Output"=w23, "Control Mode"=w74, "PhoenixMotorControlDevRef"=w72) -> ()  [unwired: 7 in, 2 out]
  n130 = disable-structure shown="Disabled" {
    disable-tunnel: w60 -> [w254 _]
    frame Disabled {
      n131 = case shown="True" w254 {
        frame False {
        }
        frame True {
          n132 = flat-sequence {
            frame #0 {
              n133 = call <vilib>:"CTRE_Phoenix_MotorControl_RefNumRegistryGet.vi"("refnum name"="Left Motor") -> ("error out"=w260:errorcluster, "PhoenixMotorControlDevRef"=w259:T11)  [unwired: 9 in]
              n134 = call <vilib>:"CTRE_Phoenix_MotorControl_RefNumRegistryGet.vi"("refnum name"="Right Motor") -> ("error out"=w266:errorcluster, "PhoenixMotorControlDevRef"=w265:T11)  [unwired: 9 in]
              n135 = call-poly <vilib>:"CTRE_Phoenix_MotorController_Get_Enhanced.vi"("PhoenixMotorControlDevRef"=w259, "error in"=w260) -> ("Position (Raw Sensor Units)"=w261:i32)  [unwired: 10 in, 3 out]
              "Left Position old" <- w261
              n136 = call-poly <vilib>:"CTRE_Phoenix_MotorController_Get_Enhanced.vi"("PhoenixMotorControlDevRef"=w265, "error in"=w266) -> ("Position (Raw Sensor Units)"=w263:i32)  [unwired: 10 in, 3 out]
              "Right Position old" <- w263
              n137 = Add(x=w261, y=20000) -> (x+y=→"Left Position New 180":i32)
              n138 = Add(x=w263, y=20000) -> (x+y=→"Right Position New 180":i32)
            }
            frame #1 {
              w276 = 0.6 ("peakOutput")
              w275 = T4 7 items=["PercentOutput"=0, "Position"=1, "Velocity"=2, "Current"=3, "Follower"=5, "MotionProfile"=6, "MotionMagic"=7, "MotionProfileArc"=10, "Disabled"=15] ("Elevator Control Mode")
              w269 = T4 7 items=["PercentOutput"=0, "Position"=1, "Velocity"=2, "Current"=3, "Follower"=5, "MotionProfile"=6, "MotionMagic"=7, "MotionProfileArc"=10, "Disabled"=15] ("Elevator Control Mode")
              # "Max Accel per 100ms"
              # "Max Cruise per 100ms"
              # "Max Accel per 100ms"
              # "Max Cruise per 100ms"
              n139 = local read "Left Position New 180"() -> (w319:i32)
              n140 = call <vilib>:"CTRE_Phoenix_MotorControl_RefNumRegistryGet.vi"("refnum name"="Right Motor") -> ("error out"=w317:errorcluster, "PhoenixMotorControlDevRef"=w316:T11)  [unwired: 9 in]
              n141 = call <vilib>:"CTRE_Phoenix_MotorControl_RefNumRegistryGet.vi"("refnum name"="Left Motor") -> ("error out"=w299:errorcluster, "PhoenixMotorControlDevRef"=w298:T11)  [unwired: 9 in]
              n142 = local read "Right Position New 180"() -> (w318:i32)
              n143 = call <vilib>:"CTRE_Phoenix_MotorControl_ConfigClosedLoopPeakOutput.vi"("error in (no error)"=w299, "peakOutput"=w276, "PhoenixMotorControlDevRef"=w298) -> ("error out"=w287:errorcluster, "PhoenixMotorControlDevRef"=w282:T11)  [unwired: 7 in]
              n144 = call <vilib>:"CTRE_Phoenix_MotorControl_ConfigClosedLoopPeakOutput.vi"("error in (no error)"=w317, "peakOutput"=w276, "PhoenixMotorControlDevRef"=w316) -> ("error out"=w305:errorcluster, "PhoenixMotorControlDevRef"=w300:T11)  [unwired: 7 in]
              n145 = call <vilib>:"CTRE_Phoenix_MotorControl_ConfigClosedLoopConstants.vi"("PhoenixMotorControlDevRef"=w282, "slotIdx"=0, "P"=0.1 ("P 2"), "I"=0.0 ("I 2"), "D"=0.0 ("D 2"), "error in (no error)"=w287, "F"=0.0 ("F 2")) -> ("PhoenixMotorControlDevRef"=w283:T11, "error out"=w288:errorcluster)  [unwired: 7 in]
              n146 = call <vilib>:"CTRE_Phoenix_MotorControl_ConfigClosedLoopConstants.vi"("PhoenixMotorControlDevRef"=w300, "slotIdx"=0, "P"=0.1 ("P 2"), "I"=0.0 ("I 2"), "D"=0.0 ("D 2"), "error in (no error)"=w305, "F"=0.0 ("F 2")) -> ("PhoenixMotorControlDevRef"=w301:T11, "error out"=w306:errorcluster)  [unwired: 7 in]
              n147 = call <vilib>:"CTRE_Phoenix_MotorControl_ConfigMotionMagic.vi"("error in (no error)"=w288, "Acceleration"="Left Max Acceleration (per 100ms)", "Cruise Velocity"="Left Cruise Velocity (per 100 ms)", "PhoenixMotorControlDevRef"=w283) -> ("error out"=w289:errorcluster, "PhoenixMotorControlDevRef"=w286:T11)  [unwired: 6 in]
              n148 = call <vilib>:"CTRE_Phoenix_MotorControl_ConfigMotionMagic.vi"("error in (no error)"=w306, "Acceleration"="Right Max Acceleration (per 100ms)", "Cruise Velocity"="Right Cruise Velocity (per 100 ms)", "PhoenixMotorControlDevRef"=w301) -> ("error out"=w307:errorcluster, "PhoenixMotorControlDevRef"=w304:T11)  [unwired: 6 in]
              n149 = To Double Precision Float(number=w319) -> (double precision float=w290:dbl)
              n150 = To Double Precision Float(number=w318) -> (double precision float=w308:dbl)
              n151 = call <vilib>:"CTRE_Phoenix_MotorControl_Set.vi"("error in (no error)"=w289, "Output"=w290, "Control Mode"=w269, "PhoenixMotorControlDevRef"=w286) -> ("error out"=w292:errorcluster, "PhoenixMotorControlDevRef"=w291:T11)  [unwired: 6 in]
              n152 = call <vilib>:"CTRE_Phoenix_MotorControl_Set.vi"("error in (no error)"=w307, "Output"=w308, "Control Mode"=w275, "PhoenixMotorControlDevRef"=w304) -> ("error out"=w310:errorcluster, "PhoenixMotorControlDevRef"=w309:T11)  [unwired: 6 in]
              n153 = call-poly <vilib>:"CTRE_Phoenix_MotorController_Get_Enhanced.vi"("PhoenixMotorControlDevRef"=w291, "error in"=w292) -> ("PhoenixMotorControlDevRef"=w293:T11, "error out"=w294:errorcluster)  [unwired: 9 in, 3 out]
              n154 = call-poly <vilib>:"CTRE_Phoenix_MotorController_Get_Enhanced.vi"("PhoenixMotorControlDevRef"=w309, "error in"=w310) -> ("PhoenixMotorControlDevRef"=w311:T11, "error out"=w312:errorcluster)  [unwired: 9 in, 3 out]
              n155 = call-poly <vilib>:"CTRE_Phoenix_MotorController_Get_Enhanced.vi"("PhoenixMotorControlDevRef"=w293, "error in"=w294) -> ("PhoenixMotorControlDevRef"=w295:T11, "Velocity (Raw Sensor Units per 100 ms)"=→"Left Velocity per 100 ms":i32, "error out"=w296:errorcluster)  [unwired: 10 in, 1 out]
              n156 = call-poly <vilib>:"CTRE_Phoenix_MotorController_Get_Enhanced.vi"("PhoenixMotorControlDevRef"=w311, "error in"=w312) -> ("PhoenixMotorControlDevRef"=w313:T11, "Velocity (Raw Sensor Units per 100 ms)"=→"Right Velocity per 100 ms":i32, "error out"=w314:errorcluster)  [unwired: 10 in, 1 out]
              n157 = call-poly <vilib>:"CTRE_Phoenix_MotorController_Get_Enhanced.vi"("PhoenixMotorControlDevRef"=w295, "error in"=w296) -> ()  [unwired: 11 in, 3 out]
              n158 = call-poly <vilib>:"CTRE_Phoenix_MotorController_Get_Enhanced.vi"("PhoenixMotorControlDevRef"=w313, "error in"=w314) -> ()  [unwired: 11 in, 3 out]
            }
          }
        }
      }
    }
    frame Enabled {
    }
  }
  n159 = call <vilib>:"CTRE_Phoenix_MotorControl_RefNumRegistryGet.vi"("refnum name"="Lift Motor") -> ("error out"=w1:errorcluster, "PhoenixMotorControlDevRef"=w2:T11)  [unwired: 9 in]
  n160 = call <vilib>:"CTRE_Phoenix_MotorControl_ConfigClosedLoopPeakOutput.vi"("error in (no error)"=w1, "peakOutput"=0.4 ("Peak Wrist Power"), "PhoenixMotorControlDevRef"=w2) -> ("error out"=w16:errorcluster, "PhoenixMotorControlDevRef"=w19:T11)  [unwired: 7 in]
  n161 = call <vilib>:"CTRE_Phoenix_MotorControl_ConfigClosedLoopConstants.vi"("PhoenixMotorControlDevRef"=w19, "slotIdx"=0, "P"=0.02 ("P 3"), "I"=0.0 ("I 3"), "D"=0.0 ("D 3"), "error in (no error)"=w16, "F"=0.0 ("F 3")) -> ("PhoenixMotorControlDevRef"=w18:T11, "error out"=w15:errorcluster)  [unwired: 7 in]
  n162 = call <vilib>:"CTRE_Phoenix_MotorControl_ConfigMotionMagic.vi"("error in (no error)"=w15, "Acceleration"=4000 ("Wrist Max Acceleration"), "Cruise Velocity"=4000 ("Wrist Cruise Velocity"), "PhoenixMotorControlDevRef"=w18) -> ("error out"=w14:errorcluster, "PhoenixMotorControlDevRef"=w17:T11)  [unwired: 6 in]
  n163 = To Double Precision Float(number="Lift Position") -> (double precision float=w13:dbl)
  n164 = call <vilib>:"CTRE_Phoenix_MotorControl_Set.vi"("error in (no error)"=w14, "Output"=w13, "Control Mode"=w4, "PhoenixMotorControlDevRef"=w17) -> ()  [unwired: 6 in, 2 out]
  n165 = call-poly <vilib>:"NT Write Value.vi"("Numeric Array"=w58, "Name"="RobotDrive Motors") -> ()  [unwired: 9 in, 1 out]
